vi "Close Master.vi"(8 "error in (no error)":errorcluster, 11 "Kasli Wrapper 2 in":refnum<class "Kasli Wrapper 2.0.lvclass">) -> (0 "error out":errorcluster, 3 "Kasli Wrapper 2 out":refnum<class "Kasli Wrapper 2.0.lvclass">)   [LabVIEW 2021, in "Kasli Wrapper 2.0.lvlib" / "Kasli Wrapper 2.0.lvclass"]
uses:
  Kasli Wrapper 2.0.lvclass
  Kasli Wrapper 2.0.lvclass/Kasli Wrapper 2.0.ctl
  38958921-fc2a-44ed-ab5c-cfcb2f248d1f.vi
  Libraries/JKI dotNET System Exec/dotnet_system_exec.lvclass
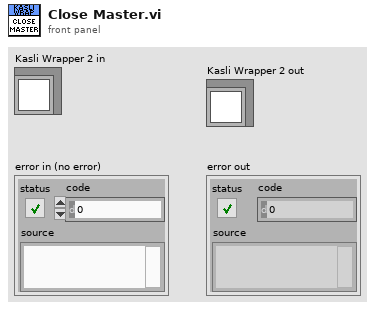
[diagram p1: front panel]
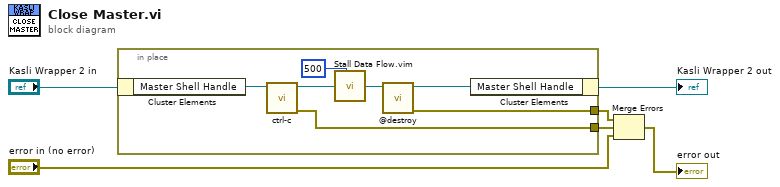
[diagram p0: block diagram]
diagram:
  n1 = in-place {
    in-place-border: [w11] -> w6
    in-place-border: [w10] -> w1
    n2 = in-place-cluster #1("Kasli Wrapper 2 in") -> ("Master Shell Handle"=w12:refnum<class "dotnet_system_exec.lvclass">)
    n3 = call "ctrl-c.vi"("dotnet_system_exec in"=w12) -> ("error out"=w11:errorcluster, "dotnet_system_exec out"=w7:refnum<class "dotnet_system_exec.lvclass">)  [unwired: 9 in]
    n4 = call "Stall Data Flow.vim"("value in"=w7, "milliseconds to wait"=u32 500) -> ("value out"=w8:refnum<class "dotnet_system_exec.lvclass">)  [unwired: 1 out]
    n5 = call-dynamic "@destroy.vi"("dotnet_system_exec in"=w8) -> ("error out"=w10:errorcluster, "dotnet_system_exec out"=w9:refnum<class "dotnet_system_exec.lvclass">)  [unwired: 9 in]
    n6 = in-place-cluster #1("Master Shell Handle"=w9) -> (→"Kasli Wrapper 2 out":refnum<class "Kasli Wrapper 2.0.lvclass">)
  }
  n7 = Merge Errors(w1, w6, "error in (no error)") -> (→"error out":errorcluster)
